vi "I and limit.vi"(6 "range":cluster{"max":dbl, "min":dbl}={"max"=100.0, "min"=-100.0}, 7 "P + D outputs":dbl, 8 "change time":dbl, 9 "I gain":dbl, 10 "integrated error":dbl, 11 "error":dbl) -> (1 "I output":dbl, 2 "integrated error":dbl, 3 "output":dbl)   [LabVIEW 2009]
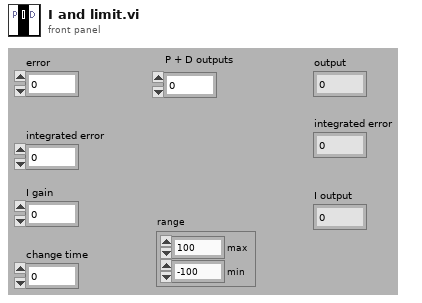
[diagram p1: front panel]
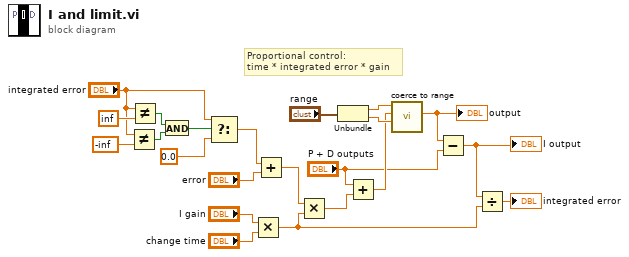
[diagram p0: block diagram]
diagram:
  # "Proportional control:\ntime * integrated error * gain"
  n1 = Not Equal?(x="integrated error", y=-inf) -> (x != y?=w16:bool)
  n2 = Not Equal?(x="integrated error", y=inf) -> (x != y?=w15:bool)
  n3 = And(x=w15, y=w16) -> (x .and. y?=w14:bool)
  n4 = Select(t="integrated error", s=w14, f=0.0) -> (s? t:f=w11:dbl)
  n5 = Multiply(x="I gain", y="change time") -> (x*y=w2:dbl)
  n6 = Add(x=w11, y="error") -> (x+y=w20:dbl)
  n7 = Multiply(x=w20, y=w2) -> (x*y=w7:dbl)
  n8 = Unbundle("range") -> ("max"=w10:dbl, "min"=w9:dbl)
  n9 = Add(x="P + D outputs", y=w7) -> (x+y=w6:dbl)
  n10 = call "coerce to range.vi"("min"=w9, "value in"=w6, "max"=w10) -> ("value out"=w5:dbl)  [unwired: 7 in, 1 out]
  "output" <- w5
  n11 = Subtract(x=w5, y="P + D outputs") -> (x-y=w3:dbl)
  "I output" <- w3
  n12 = Divide(x=w3, y=w2) -> (x/y=→"integrated error":dbl)
